vi "descramble.vi"(2 "scrambled":string) -> (6 "OUT":string)   [LabVIEW 2020]
doc: "Decode scrambled data"
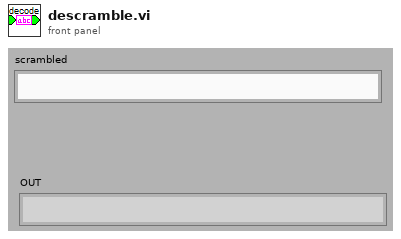
[diagram p1: front panel]
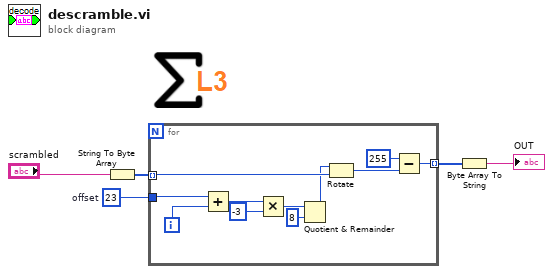
[diagram p0: block diagram]
diagram:
  w3 = 23  # offset
  n1 = String To Byte Array(string="scrambled") -> (unsigned byte array=w4:u8[])
  n2 = for {
    tunnel: w3 -> [w16]
    tunnel: w4 -> [w9] mode=indexing
    tunnel: [w6] -> w5 mode=indexing
    i -> [w15]
    n3 = Add(x=w16, y=w15) -> (x+y=w13:i32)
    n4 = Multiply(x=w13, y=-3) -> (x*y=w11:i32)
    n5 = Quotient & Remainder(x=w11, y=8) -> (x-y*floor(x/y)=w8:i32)  [unwired: 1 out]
    n6 = Rotate(1:w9, 2:w8) -> (0:w7:u8)
    n7 = Subtract(x=u8 255, y=w7) -> (x-y=w6:u8)
  }
  n8 = Byte Array To String(unsigned byte array=w5) -> (string=→"OUT":string)
